vi "Login(BoardPort).vi"(8 "error in (no error)":errorcluster, 10 "SrvName (local)":string="local", 11 "resource in":T1) -> (0 "error out":errorcluster, 2 "Handle":u32, 3 "resource out":T1)   [LabVIEW 2020, in "AIM664LV.lvlib"]
uses:
  AIM664LV.lvlib
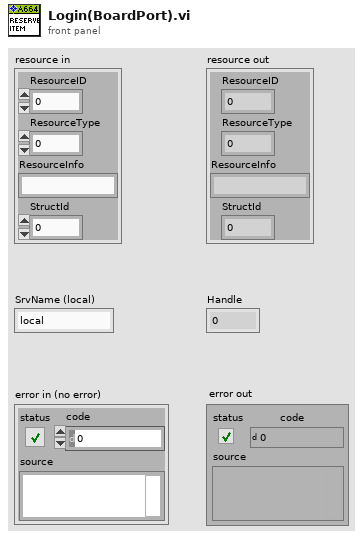
[diagram p1: front panel]
types:
  T1 = cluster{"ResourceID":u32, "ResourceType":u32, "ResourceInfo":string, "StructId":u32}
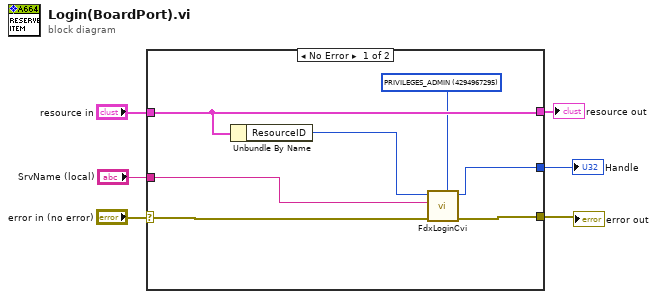
[diagram p0: block diagram]
diagram:
  n1 = case shown="No Error" "error in (no error)" {
    selector: "error in (no error)" -> [w13 w14]
    tunnel: "resource in" -> [w10 _]
    tunnel: [w12 w14] -> w4
    tunnel: [w11 _] -> w3
    tunnel: [w10 _] -> w2
    tunnel: "SrvName (local)" -> [w8 _]
    frame No Error {
      w7 = u32 4294967295 items=["PRIVILEGES_ADMIN"=4294967295] ("Privileges")
      n2 = Unbundle By Name(w10) -> ("ResourceID"=w9:u32)
      n3 = call "FdxLoginCvi.vi"("Privileges"=w7, "error in"=w13, "SrvName"=w8, "ResourceID"=w9) -> ("error out"=w12:errorcluster, "InstrumentHandle"=w11:u32)  [unwired: 6 in]
    }
    frame Error {
    }
  }
  "error out" <- w4
  "Handle" <- w3
  "resource out" <- w2
